vi "Servo Open.vi"(8 "Error In":errorcluster, 10 "Channels":u8[](array[numeric]), 11 "LINX Device Config":T1) -> (0 "Error Out":errorcluster, 3 "LINX Device Config":T1)   [LabVIEW 2019, in "LMH-LINX.lvlib" / "Device.lvlib"]
uses:
  <vilib>/MakerHub/LINX/Private/Device/Device.lvlib
  <vilib>/MakerHub/LINX/Private/Device/Type Defs/LINX Device Config.ctl
  <vilib>/MakerHub/LINX/Private/Type Defs/Interface.ctl
  <vilib>/MakerHub/LINX/Private/Device/Type Defs/TCP Config.ctl
  <vilib>/MakerHub/LINX/Private/Device/Type Defs/Channels.ctl
  <vilib>/MakerHub/LINX/Private/Type Defs/Error Type.ctl
  <vilib>/MakerHub/LINX/LMH-LINX.lvlib
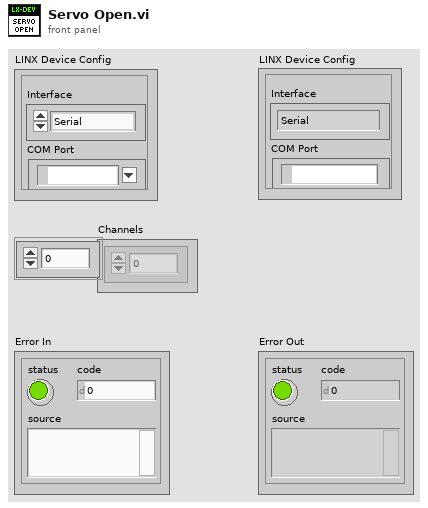
[diagram p1: front panel]
types:
  T1 = typedef "LMH-LINX.lvlib/Device.lvlib/LINX Device Config.ctl" = cluster{"Interface":T2, "COM Port":refnum<visa-resource-name>, "TCP Configuration":T3, "Device Family":u8, "Device ID":u8, "Device Name":string, "TCP Ref":refnum<k5>, "Channels":T4}
  T2 = typedef "LMH-LINX.lvlib/Interface.ctl" = enum16{"Serial", "TCP"}
  T3 = typedef "LMH-LINX.lvlib/Device.lvlib/TCP Config.ctl" = cluster{"IP Address":string, "Port":u16}
  T4 = typedef "LMH-LINX.lvlib/Channels.ctl" = cluster{"DI":u8[], "DO":u8[], "AI":u8[], "AO":u8[], "PWM":u8[], "QE":u8[], "UART":u8[], "I2C 2":u8[], "SPI":u8[], "CAN":u8[], "Servo":u8[], "AI Ref (V)":dbl, "AI Resolution (Bits)":u8, "AO Ref (V)":dbl, "AO Resolution (Bits)":u8}
  T5 = typedef "LMH-LINX.lvlib/Error Type.ctl" = enum16{"Unknown", "Timeout", "Corrupt Return Packet", "Unable To Connect", "Command Not Supported", "Channel DNE", "Invalid COM Config", "Firmware Version Mismatch", "myRIO Support", "CMD Specific Error", "Local IO Not Supported"}
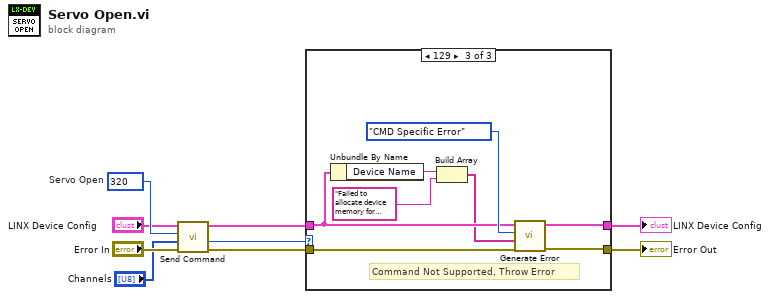
[diagram p0: block diagram]
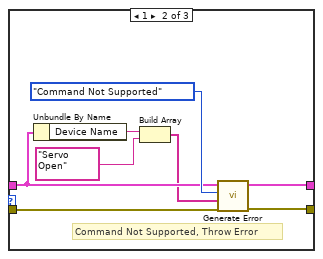
[diagram p3: hidden frame]
diagram:
  w8 = u16 320  # Servo Open
  n1 = call <vilib>:"Send Command.vi"("Error In"="Error In", "ARGS"="Channels", "CMD"=w8, "LINX Device Config"="LINX Device Config") -> ("Error Out"=w3:errorcluster, "Status"=w1:u8, "LINX Device Config"=w5:T1)  [unwired: 4 in, 1 out]
  n2 = case shown="129" w1 {
    tunnel: [w11 w17 w25] -> w6
    tunnel: w5 -> [w11 w13 w21]
    tunnel: [w10 w18 w26] -> w4
    tunnel: w3 -> [w10 w19 w27]
    frame 0, Default {
      # "Status OK, Process Data"
    }
    frame 1 {
      # "Command Not Supported, Throw Error"
      n3 = Unbundle By Name(w13) -> ("Device Name"=w15:string)
      n4 = Build Array(w15, "Servo Open") -> (w12:string[])
      n5 = call <vilib>:"Generate Error.vi"("Error In"=w19, "Arguments"=w12, "Error Type"=Error_Type."Command Not Supported", "LINX Device Config"=w13) -> ("Error Out"=w18:errorcluster, "Dup LINX Device Config"=w17:T1)  [unwired: 6 in]
    }
    frame 129 {
      # "Command Not Supported, Throw Error"
      n6 = Unbundle By Name(w21) -> ("Device Name"=w23:string)
      n7 = Build Array(w23, "Failed to allocate device memory for servo object.") -> (w20:string[])
      n8 = call <vilib>:"Generate Error.vi"("Error In"=w27, "Arguments"=w20, "Error Type"=Error_Type."CMD Specific Error", "LINX Device Config"=w21) -> ("Error Out"=w26:errorcluster, "Dup LINX Device Config"=w25:T1)  [unwired: 6 in]
    }
  }
  "Error Out" <- w4
  "LINX Device Config" <- w6
